vi "Configure Port.vi"(8 "error in (no error)":errorcluster, 10 "Port Function (0:Trigger)":u16(ring) items=["Trigger", "RIDF", "Digital I/O"], 11 "VISA resource name":refnum<visa-resource-name>) -> (0 "error out":errorcluster, 3 "VISA resource name out":refnum<visa-resource-name>)   [LabVIEW 2021, in "Keithley 2200 Series.lvlib"]
doc: "Sets the mode of the port for the power supply."
uses:
  <instrlib>/Keithley 2200 Series/Keithley 2200 Series.lvlib
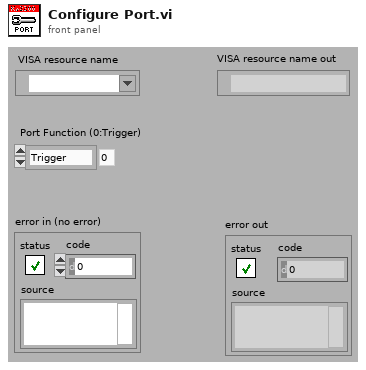
[diagram p1: front panel]
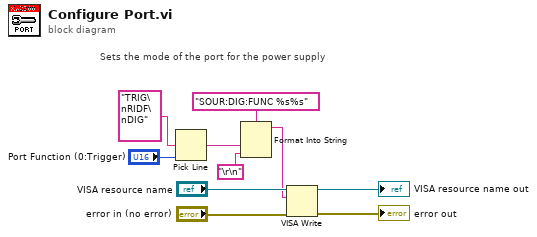
[diagram p0: block diagram]
diagram:
  # "Sets the mode of the port for the power supply"
  n1 = Pick Line(multi-line string="TRIG\nRIDF\nDIG" ("string (\"\")"), line index="Port Function (0:Trigger)") -> (output string=w4:string)  [unwired: 1 out]
  n2 = Format Into String(format string="SOUR:DIG:FUNC %s%s", w4, "\r\n" ("End of Line Constant")) -> (resulting string=w1:string)  [unwired: 2 in, 1 out]
  n3 = VISA Write(VISA resource name="VISA resource name", write buffer=w1, error in (no error)="error in (no error)") -> (VISA resource name out=→"VISA resource name out":refnum<visa-resource-name>, error out=→"error out":errorcluster)  [unwired: 1 out]
